vi "svfa_Spectrum Peak Tone Search and Estimation (magnitude).vi"(7 "spectrum includes end points?":bool, 8 "error in (no error)":errorcluster, 9 "criterion":T1={"Single/Multiple"=enum."Single Max Peak", "Threshold"=-1.0, "advanced search"={"approx freq. (optional)"=-1.0, "search (+/- % of Fsampl.)"=5.0}} {"advanced search"."search (+/- % of Fsampl.)" format="%0.2p"; "advanced search"."approx freq. (optional)" format="%0.2p"; "Threshold" format="%.2f"}, 10 "spectrum info":T3={"channel name"="", "description"="", "x-axis units"=0, "spectral info"={"spectrum type"=enum."Power [Magnitude^2]", "linear/dB"=enum."linear", "window"=0, "window size"=0, "FFT size"=0}, "engineering units"=0, "custom label"="", "dB reference [EU]"=0.0, "peak units"=enum."rms", "weighting filter"=0, "spectral density?"=FALSE, "unit label"="", "spectrum skewed?"=FALSE, "complimentary spectrum units"=enum."none"} {"x-axis units" items=["Time (s)"=0, "Frequency-CB (Hz)"=1, "Frequency-CPB (Hz)"=1248, "Frequency-Arbitrary (Hz)"=2357, "Quefrency (s)"=2, "Revolutions (rev)"=3, "Order"=4, "Speed (RPM)"=11, "Speed (rad/s)"=21, "Index"=65535]; "weighting filter" items=["Linear", "A-weighting", "B-weighting", "C-weighting", "ITU-R 468-4", "Dolby", "CCITT", "C-message", "Wb", "Wc", "Wd", "We", "Wf", "Wh", "Wj", "Wk", "Wm", "AES17 20 kHz lowpass", "AES17 40 kHz lowpass", "AES17 20 kHz highpass", "AES17 40 kHz highpass"]; "dB reference [EU]" format="%.2f"; "engineering units" items=["custom..."=0, "V"=1, "A"=21, "C"=30, "pC"=31, "s"=32, "-"=29, "Pa"=2, "N"=20, "g"=3, "m/s^2"=4, "m/s"=5, "m"=6, "mm/s"=12, "mm"=13, "micron/s"=14, "micron"=15, "in/s^2"=7, "in/s"=8, "in"=9, "mil/s"=10, "mil"=11, "rad/s^2"=16, "rad/s"=17, "rad"=18, "deg/s^2"=26, "deg/s"=27, "deg"=28, "RPM"=22, "cycle/s^2"=23, "Hz"=24, "cycle"=25, "strain"=19]; "spectral info"."window" items=["None "=0, "Hanning"=1, "Hamming"=2, "Blackman-Harris"=3, "Exact Blackman"=4, "Blackman"=5, "Flat Top"=6, "4 Term B-Harris "=7, "7 Term B-Harris"=8, "Low Sidelobe"=9, "Force - Exponential"=10, "Gaussian"=62]}, 11 "power/amplitude spectrum":cluster{"f0":dbl, "df":dbl, "spectrum":dbl[]}={"f0"=0.0, "df"=1.0, "spectrum"=[]} {"spectrum" format="%.2f"; "df" format="%.2f"; "f0" format="%.2f"}) -> (0 "error out":errorcluster, 2 "Number of peaks":i32, 3 "peaks":T2(array[cluster]) {"phase [degree]" format="%.2f"; "value" format="%.2f"; "frequency [Hz]" format="%.2f"})   [LabVIEW 2017]
uses:
  <vilib>/addons/_NISVFA/_Shared subVIs/Controls/svc_Spectrum Info.ctl
  <vilib>/addons/_NISVFA/_Shared subVIs/Controls/svc_X-Axis Units.ctl
  <vilib>/addons/_NISVFA/_Shared subVIs/Controls/svc_Spectrum Type.ctl
  <vilib>/addons/_NISVFA/_Shared subVIs/Controls/svc_Engineering Units Text Ring.ctl
  <vilib>/addons/_NISVFA/_Shared subVIs/Controls/svc_Weighting Filter Text Ring.ctl
  <vilib>/addons/_NISVFA/_Shared subVIs/Controls/svc_Complimentary Spectrum Units.ctl
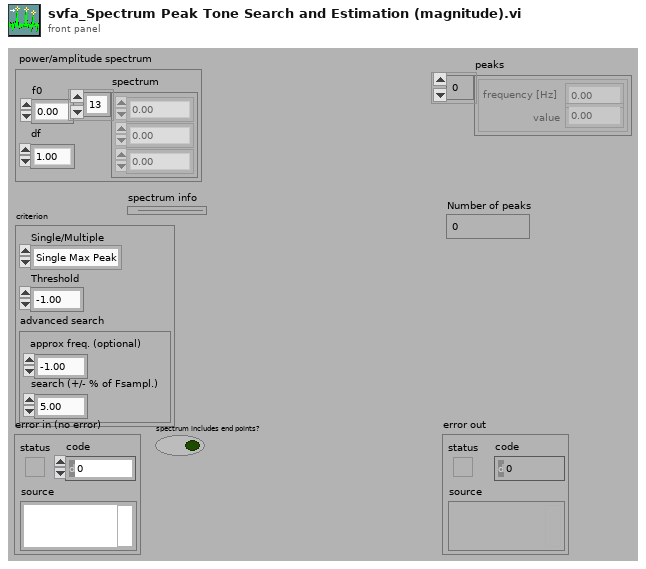
[diagram p1: front panel]
types:
  T1 = cluster{"Single/Multiple":enum16{"Multiple Peaks", "Single Max Peak"}, "Threshold":dbl, "advanced search":cluster{"approx freq. (optional)":dbl, "search (+/- % of Fsampl.)":dbl}}
  T2 = cluster{"frequency [Hz]":dbl, "value":dbl, "phase [degree]":dbl}[]
  T3 = typedef "svc_Spectrum Info.ctl" = cluster{"channel name":string, "description":string, "x-axis units":T4, "spectral info":cluster{"spectrum type":T5, "linear/dB":enum16{"linear", "dB"}, "window":u16, "window size":i32, "FFT size":i32}, "engineering units":T6, "custom label":string, "dB reference [EU]":dbl, "peak units":enum16{"rms", "peak", "peak-peak"}, "weighting filter":T7, "spectral density?":bool, "unit label":string, "spectrum skewed?":bool, "complimentary spectrum units":T8}
  T4 = typedef "svc_X-Axis Units.ctl" = u16
  T5 = typedef "svc_Spectrum Type.ctl" = enum16{"FFT Spectrum [complex]", "Amplitude [Magnitude]", "Power [Magnitude^2]", "Cross Spectrum [complex]", "Frequency Response [Complex]"}
  T6 = typedef "svc_Engineering Units Text Ring.ctl" = u16
  T7 = typedef "svc_Weighting Filter Text Ring.ctl" = u16
  T8 = typedef "svc_Complimentary Spectrum Units.ctl" = enum16{"none", "radians", "degrees", "cycles", "imaginary"}
  T9 = cluster{"frequency [Hz]":dbl, "amplitude":dbl, "phase [degree]":dbl}
  T10 = cluster{"frequency [Hz]":dbl, "amplitude":dbl, "phase [degree]":dbl}[]
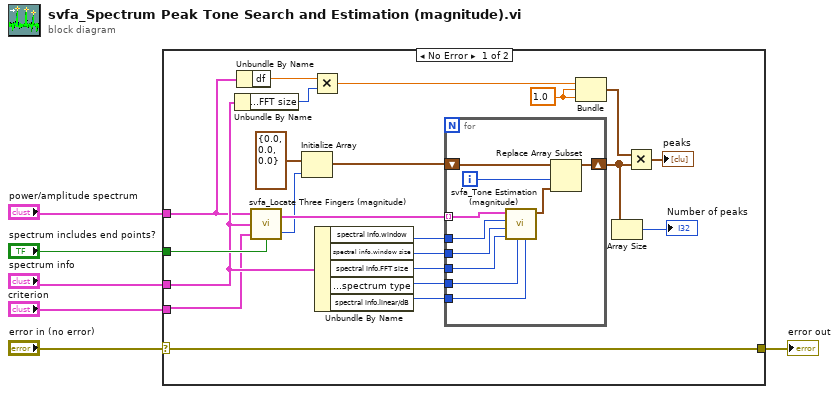
[diagram p0: block diagram]
diagram:
  n1 = case shown="No Error" "error in (no error)" {
    selector: "error in (no error)" -> [w11 w39]
    tunnel: [w11 w39] -> w5
    tunnel: "spectrum info" -> [w15 _]
    tunnel: "criterion" -> [w13 _]
    tunnel: "power/amplitude spectrum" -> [w14 _]
    tunnel: "spectrum includes end points?" -> [w16 _]
    frame No Error {
      w23 = 1.0 ("x*y")
      n2 = Unbundle By Name(w15) -> ("spectral info.FFT size"=w20:i32)
      n3 = Unbundle By Name(w14) -> ("df"=w21:dbl)
      n4 = call <vilib>:"svfa_Locate Three Fingers (magnitude).vi"("spectrum includes end points?"=w16, "criterion"=w13, "spectrum info"=w15, "spectrum"=w14) -> ("number of tones"=w24:i32, "three fingers (frequency normalized)"=w28:cluster{"f0":dbl, "df":dbl, "spectrum":dbl[]}[])
      n5 = Initialize Array(T9 {"frequency [Hz]"=0.0, "amplitude"=0.0, "phase [degree]"=0.0} ("single tone info."), w24) -> (w25:T10)
      n6 = Multiply(x=w21, y=w20) -> (x*y=w22:dbl)
      n7 = Unbundle By Name(w15) -> ("spectral info.window"=w10:u16, "spectral info.window size"=w9:i32, "spectral info.FFT size"=w8:i32, "spectral info.spectrum type"=w12:T5, "spectral info.linear/dB"=w7:enum16{"linear", "dB"})
      n8 = for {
        tunnel: w28 -> [w35] mode=indexing
        shift-right: [w38] -> w17
        shift-left: w25 -> [w34]
        tunnel: w12 -> [w33]
        tunnel: w10 -> [w32]
        tunnel: w9 -> [w31]
        tunnel: w8 -> [w30]
        tunnel: w7 -> [w29]
        i -> [w36]
        n9 = call <vilib>:"svfa_Tone Estimation (magnitude).vi"("linear/dB"=w29, "spectrum type"=w33, "FFT size"=w30, "window size"=w31, "window"=w32, "three fingers"=w35) -> ("single tone info."=w37:T9)  [unwired: 5 in]
        n10 = Replace Array Subset(array=w34, new element=w37, index=w36) -> (w38:T10)
      }
      n11 = Bundle(w22, "x*y"=w23, "x*y"=w23) -> (w18:cluster{dbl, "x*y":dbl, "x*y":dbl})  [unwired: 1 in]
      n12 = Array Size(array=w17) -> (size(s)=→"Number of peaks":i32)
      n13 = Multiply(x=w18, y=w17) -> (x*y=→"peaks":cluster{dbl, dbl, dbl}[])
    }
    frame Error {
    }
  }
  "error out" <- w5
